vi "writeValveSetpoints.vi"(8 "error in (no error)":errorcluster, 10 "ILC in":refnum<class "ILC.lvclass">, 11 "IActuatorCylinder in":refnum<class "IActuatorCylinder.lvclass">) -> (0 "error out":errorcluster, 2 "ILC out":refnum<class "ILC.lvclass">, 3 "IActuatorCylinder out":refnum<class "IActuatorCylinder.lvclass">)   [LabVIEW 2015, in "IActuatorCylinder.lvclass"]
uses:
  IActuatorCylinder.lvclass
  <userlib>/Common/ILC/ILC/ILC.lvclass
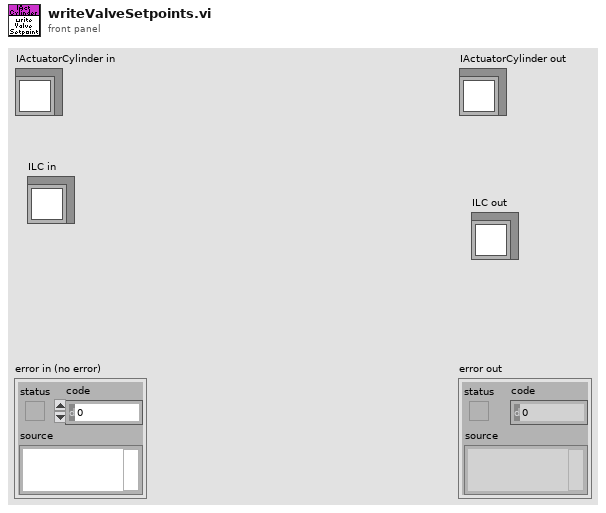
[diagram p1: front panel]
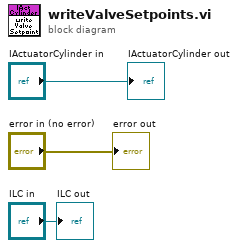
[diagram p0: block diagram]
diagram:
  "error out" <- "error in (no error)"
  "IActuatorCylinder out" <- "IActuatorCylinder in"
  "ILC out" <- "ILC in"
